vi "CursorPositionSet.vi"(8 "error in (no error)":errorcluster, 10 "CursorPosition":cluster{"x":i16, "y":i16}, 11 "Gviewer in":refnum<class "Gviewer.lvclass">) -> (0 "error out":errorcluster, 3 "Gviewer out":refnum<class "Gviewer.lvclass">)   [LabVIEW 2020, in "Sgraph_lib_V1.lvlib" / "Gviewer.lvclass"]
doc: "Andre Koelewijn, 6 feb 2022\n\nWrite the cursor position that was set when hovering over the graph in cursor mode."
uses:
  Gviewer.lvclass
  Gviewer.lvclass/Gviewer.ctl
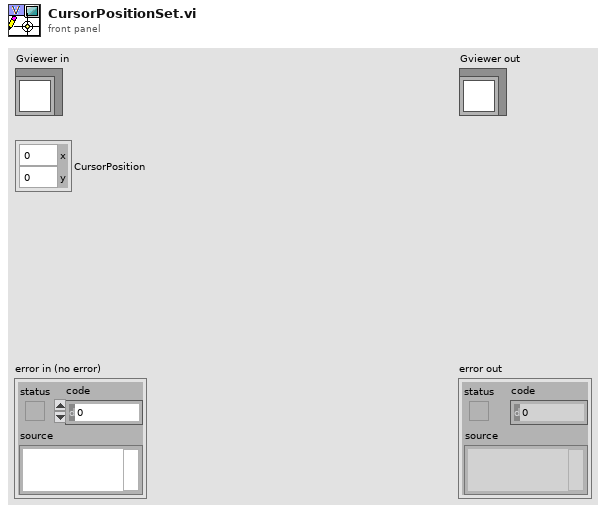
[diagram p1: front panel]
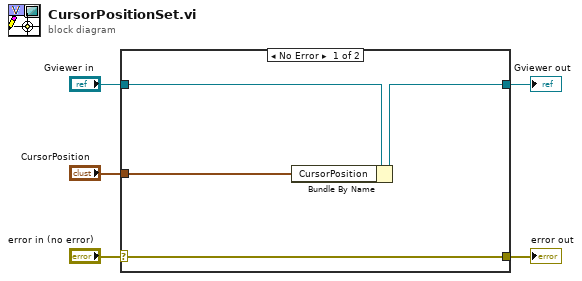
[diagram p0: block diagram]
diagram:
  n1 = case shown="No Error" "error in (no error)" {
    selector: "error in (no error)" -> [w9 w10]
    tunnel: [w9 w10] -> w4
    tunnel: [w7 w11] -> w2
    tunnel: "Gviewer in" -> [w8 w11]
    tunnel: "CursorPosition" -> [w6 _]
    frame No Error {
      n2 = Bundle By Name(cluster=w8, "CursorPosition"=w6) -> (w7:refnum<class "Gviewer.lvclass">)
    }
    frame Error {
    }
  }
  "error out" <- w4
  "Gviewer out" <- w2
